vi "WFS Self-Test.vi"(8 "error in (no error)":errorcluster {"code" format="%.0x"}, 11 "instrument handle":refnum<visa-resource-name>) -> (0 "error out":errorcluster {"code" format="%.0x"}, 1 "Self-Test Message":string, 2 "Self Test Result":i16 format="%.0g", 3 "instrument handle out":refnum<visa-resource-name>)   [LabVIEW 2020]
doc: "This VI causes the instrument to perform a self-test and returns the result of that self-test."
uses:
  WFS_32.dll
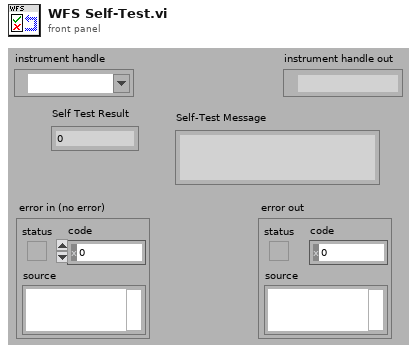
[diagram p1: front panel]
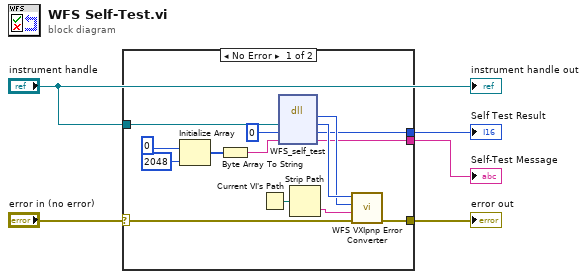
[diagram p0: block diagram]
diagram:
  n1 = case shown="No Error" "error in (no error)" {
    selector: "error in (no error)" -> [w11 w20]
    tunnel: [w10 w20] -> w4
    tunnel: "instrument handle" -> [w8 _]
    tunnel: [w7 _] -> w2
    tunnel: [w6 _] -> w1
    frame No Error {
      n2 = Initialize Array(u8 0, 2048 ("size of self-test message")) -> (w18:u8[])
      n3 = Byte Array To String(unsigned byte array=w18) -> (string=w17:string)
      n4 = Current VI's Path() -> (path=w16:path)
      n5 = dll-call lib="WFS_*.*" fn="WFS_self_test"("instrument handle"=w8, "self test result"=i16 0, "self-test message"=w17) -> ("Status"=w13:i32, "instrument handle"=w14:u32, "self test result"=w7:i16, "self-test message"=w6:string)  [unwired: 3 in, 2 out]
      n6 = Strip Path(path=w16) -> (name=w12:string)  [unwired: 1 out]
      n7 = call "WFS VXIpnp Error Converter.vi"("error in (no error)"=w11, "Name Of VI (\"\")"=w12, "CVI Error Code (0)"=w13, "instrument handle"=w14) -> ("error out"=w10:errorcluster)  [unwired: 6 in, 1 out]
    }
    frame Error {
    }
  }
  "error out" <- w4
  "Self Test Result" <- w2
  "Self-Test Message" <- w1
  "instrument handle out" <- "instrument handle"
